vi "Render.vi"(8 "error in (no error)":errorcluster, 10 "String in":string, 11 "Bold in":refnum<class "Code.lvclass">) -> (0 "error out":errorcluster, 2 "String out":string, 3 "Bold out":refnum<class "Code.lvclass">)   [LabVIEW 2021, in "Markdown.lvlib" / "Code.lvclass"]
uses:
  Code.lvclass
  C:/GitHub/Markdown/src/Markdown/Markdown.lvclass
  GetCodeTag.vi
  Code.lvclass/Code.ctl
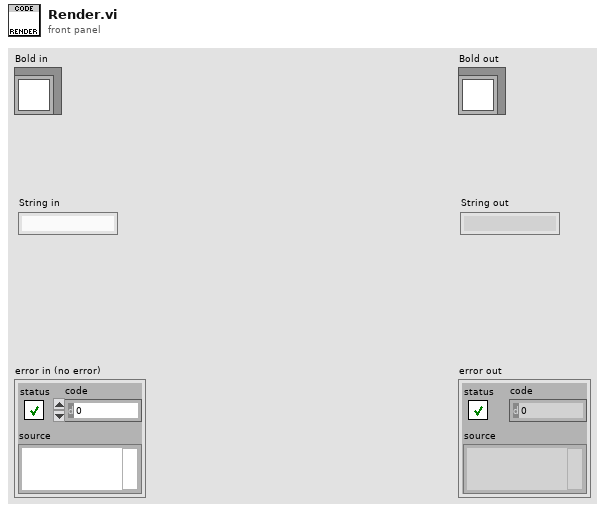
[diagram p1: front panel]
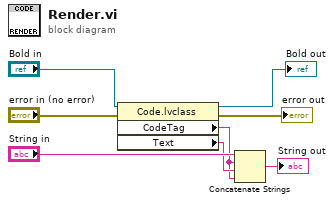
[diagram p0: block diagram]
diagram:
  n1 = property class="Code.lvclass"(reference="Bold in", error in="error in (no error)") -> (reference out=→"Bold out":refnum<class "Code.lvclass">, error out=→"error out":errorcluster, "CodeTag"=w6:string, "Text"=w7:string)
  n2 = Concatenate Strings("String in", w6, w7, w6) -> (→"String out":string)
